vi "Delete Position from File.vi"(1 "index":i32, 3 "error in":errorcluster) -> (7 "positions":T1[](array[typedef]), 10 "error out":errorcluster)   [LabVIEW 2020, in "Manipulator.lvlib"]
uses:
  Manipulator.lvlib
  Named Position.ctl
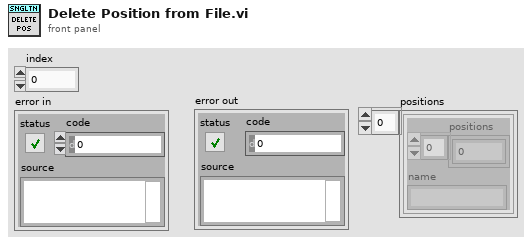
[diagram p1: front panel]
types:
  T1 = typedef "Manipulator.lvlib/Named Position.ctl" = cluster{"positions":dbl[], "name":string}
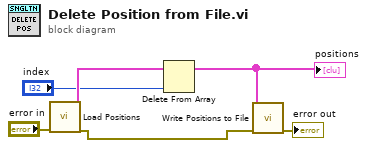
[diagram p0: block diagram]
diagram:
  n1 = call "Load Positions.vi"("error in"="error in") -> ("error out"=w3:errorcluster, "positions"=w6:T1[])  [unwired: 9 in]
  n2 = Delete From Array(array=w6, index="index") -> (array with subset deleted=w4:T1[])  [unwired: 1 in, 1 out]
  "positions" <- w4
  n3 = call "Write Positions to File.vi"("error in (no error)"=w3, "positions"=w4) -> ("error out"=→"error out":errorcluster)  [unwired: 9 in]
